vi "Angle Distance.vi"(1 "Target Angle":dbl(knob) scale=-180.0..180.0, 2 "Current Angle":dbl(knob) scale=-180.0..180.0) -> (0 "Distance":dbl)   [LabVIEW 2018]
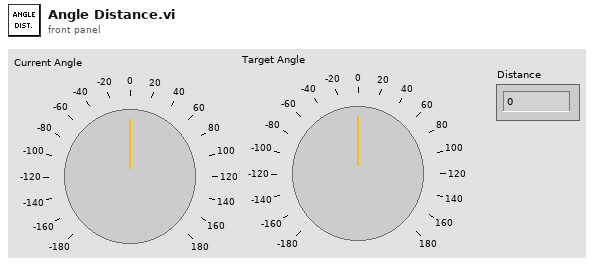
[diagram p1: front panel]
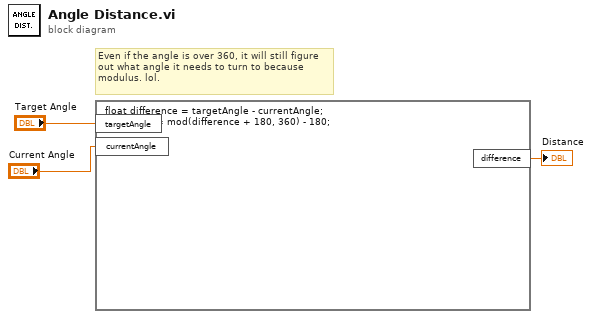
[diagram p0: block diagram]
diagram:
  # "Even if the angle is over 360, it will still figure\nout what angle it needs to turn to because \nmodulus. lol."
  n1 = formula code="float difference = targetAngle - currentAngle;\ndifference = mod(difference + 180, 360) - 180;"("targetAngle"="Target Angle", "currentAngle"="Current Angle") -> ("difference"=→"Distance":dbl)
